vi "KalmanforRelX,Y,angle_171213.vi"(8 "i":i32, 9 "angle":sgl, 10 "RelY":sgl, 11 "RelX":sgl) -> (1 "nextangle":dbl, 2 "nextY":dbl, 3 "nextX":dbl)   [LabVIEW 2016]
uses:
  Globaltracker.vi
panel:
  out "old angle":sgl
  out "old Y":sgl
  out "old X":sgl
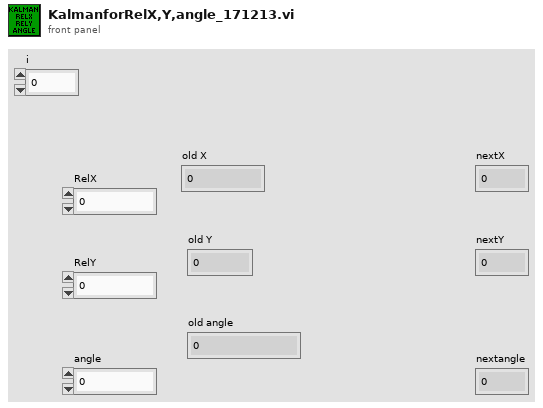
[diagram p1: front panel]
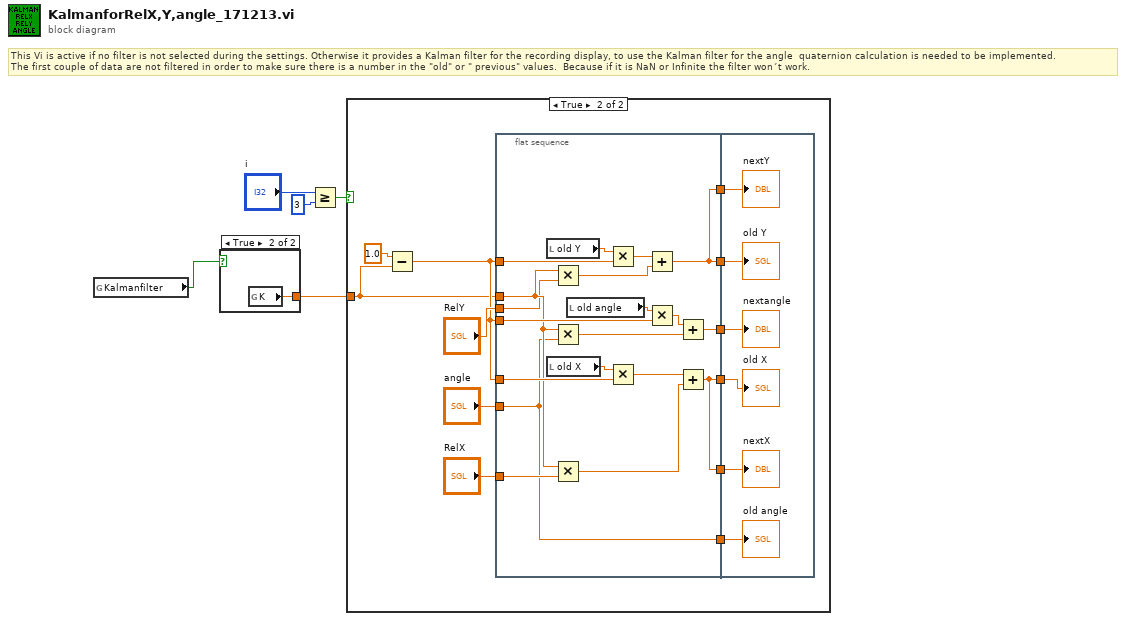
[diagram p0: block diagram]
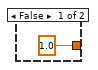
[diagram p2: hidden frame]
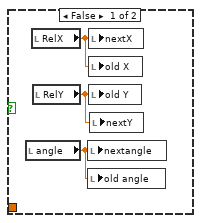
[diagram p3: hidden frame]
diagram:
  # "This Vi is active if no filter is not selected during the settings. Otherwise it provides a Kalman filter for the recording display, to use the Kalman filter for the angle  quaternion calculation is needed to be implemented.\nThe first couple of data are not filtered in order to make sure there is a number in the \"old\" or \" previous\" values.  Because if it is NaN or Infinite the filter won´t work."
  n1 = global read "Globaltracker.vi" "Kalmanfilter"() -> (w2:bool)
  n2 = case shown="True" w2 {
    tunnel: [1.0 ("K") w7] -> w1
    frame False {
    }
    frame True {
      n3 = global read "Globaltracker.vi" "K"() -> (w7:dbl)
    }
  }
  n4 = Greater Or Equal?(x="i", y=3 ("x")) -> (x >= y?=w3:bool)
  n5 = case shown="True" w3 {
    tunnel: w1 -> [_ w11]
    frame False {
      n6 = local read "angle"() -> (w8:sgl)
      n7 = local read "RelX"() -> (w10:sgl)
      n8 = local read "RelY"() -> (w9:sgl)
      n9 = local write "nextangle"(w8) -> ()
      n10 = local write "old angle"(w8) -> ()
      n11 = local write "nextX"(w10) -> ()
      n12 = local write "old X"(w10) -> ()
      n13 = local write "old Y"(w9) -> ()
      n14 = local write "nextY"(w9) -> ()
    }
    frame True {
      n15 = Subtract(x=1.0, y=w11) -> (x-y=w15:dbl)
      n16 = flat-sequence {
        tunnel: "RelX" -> [w31]
        tunnel: w11 -> [w32]
        tunnel: "RelY" -> [w30]
        tunnel: [w25] -> w20
        tunnel: "angle" -> [w25]
        tunnel: [w23] -> w18
        tunnel: [w24] -> w17
        tunnel: w15 -> [w40]
        tunnel: w15 -> [w36]
        tunnel: w15 -> [w33]
        tunnel: [w23] -> w14
        tunnel: [w24] -> w13
        tunnel: [w27] -> w12
        tunnel: w20 -> [w47]
        tunnel: w18 -> [w43]
        tunnel: w17 -> [w44]
        tunnel: w14 -> [w46]
        tunnel: w13 -> [w45]
        tunnel: w12 -> [w42]
        frame #0 {
          n17 = local read "old Y"() -> (w28:sgl)
          n18 = local read "old X"() -> (w29:sgl)
          n19 = Multiply(x=w32, y=w30) -> (x*y=w37:dbl)
          n20 = Multiply(x=w32, y=w25) -> (x*y=w35:dbl)
          n21 = Multiply(x=w32, y=w31) -> (x*y=w41:dbl)
          n22 = local read "old angle"() -> (w26:sgl)
          n23 = Multiply(x=w28, y=w36) -> (x*y=w38:dbl)
          n24 = Multiply(x=w29, y=w40) -> (x*y=w39:dbl)
          n25 = Add(x=w38, y=w37) -> (x+y=w23:dbl)
          n26 = Multiply(x=w26, y=w33) -> (x*y=w34:dbl)
          n27 = Add(x=w34, y=w35) -> (x+y=w27:dbl)
          n28 = Add(x=w39, y=w41) -> (x+y=w24:dbl)
        }
        frame #1 {
          "old X" <- w44
          "old Y" <- w43
          "old angle" <- w47
          "nextX" <- w45
          "nextY" <- w46
          "nextangle" <- w42
        }
      }
    }
  }
